vi "clear Error.vi"   [LabVIEW 2012, in "cvlib.lvlib"]
doc: "extern \"C\" __declspec(dllexport) void __cdecl clearError();"
uses:
  cvlib.lvlib
  cvlib.dll
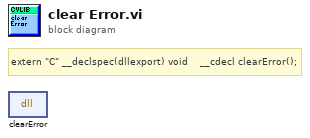
[diagram p0: block diagram]
diagram:
  # "extern \"C\" __declspec(dllexport) void \t\t\t__cdecl clearError();"
  n1 = dll-call lib="C:/Users/myerslab/workspace2/Libraries/ClearVolume/cpp/labview/lvcvlib/cvlib.*" fn="clearError"() -> ()  [unwired: 4 in, 2 out]
